vi "Robot Global Data.vi"() -> ()   [LabVIEW 2014]
doc: "This global VI can contain as many global variables as you need. Place a control on the panel, give it a good name. To read or write to it from a VI, drag the icon to the diagram of that VI. You can also drag from the project. Click on the node to change which global you access. You shouldn't have multiple locations writing to a global or it will cause a race-condition."
uses:
  <vilib>/Rock Robotics/WPI/Camera/WPI_CameraImageSize.ctl
  <vilib>/Rock Robotics/WPI/DriverStation/WPI_DriverStationRobotMode2.ctl
panel:
  in  "Tele Times":cluster{"X":dbl[], "Y":dbl[]}
  out "Doors Oper":bool
  in  "String Lift":T1
  in  "NavX":cluster{"Update Speed (Hz)":dbl, "Turn":dbl}
  out "Dashboard Cluster":T2
  in  "Tote Cluster":T3
  out "Recycling Can Cluster":T4
  in  "Drive Cluster":cluster{"A":dbl, "B":dbl, "R":dbl, "Gyro":dbl}
  in  "Robot Mode":T5
  in  "image size":T6=enum."320x240"
  in  "Enable Vision":bool
  # "Unused:"
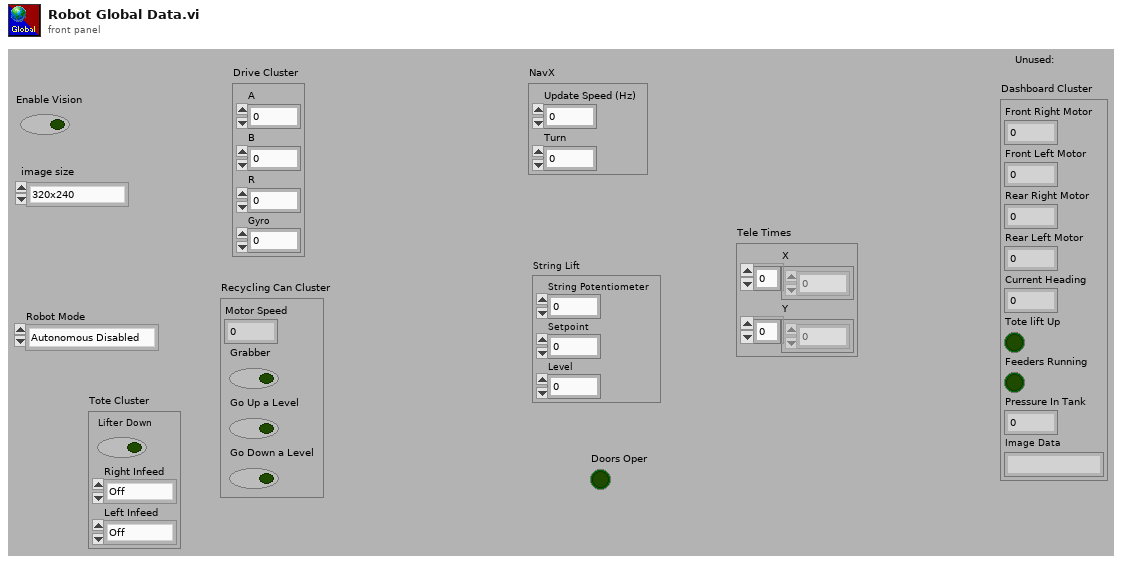
[diagram p1: front panel]
types:
  T1 = cluster{"String Potentiometer":dbl, "Setpoint":dbl, "Level":sgl}
  T2 = cluster{"Front Right Motor":dbl, "Front Left Motor":dbl, "Rear Right Motor":dbl, "Rear Left Motor":dbl, "Current Heading":dbl, "Tote lift Up":bool, "Feeders Running":bool, "Pressure In Tank":dbl, "Image Data":string}
  T3 = cluster{"Lifter Down":bool, "Right Infeed":enum16{"Off", "Forward", "Reverse"}, "Left Infeed":enum16{"Off", "Forward", "Reverse"}}
  T4 = cluster{"Motor Speed":dbl, "Grabber":bool, "Go Up a Level":bool, "Go Down a Level":bool}
  T5 = typedef "WPI_DriverStationRobotMode2.ctl" = enum16{"Autonomous Disabled", "Autonomous Enabled", "Teleop Disabled", "Teleop Enabled", "Disconnected", "Finish", "Test Disabled", "Test Enabled", "Emergency Stopped"}
  T6 = typedef "WPI_CameraImageSize.ctl" = enum16{"640x480", "320x240", "160x120", "Custom"}
diagram:
